vi "simx Set Vision Sensor Image.vi"(5 "operationMode":i32, 6 "options":u8, 7 "bufferSize":i32, 8 "error in (no error)":errorcluster, 9 "image":string, 10 "sensorHandle":i32, 11 "clientID":i32) -> (0 "error out":errorcluster, 1 "image out":string, 3 "function return":i32)   [LabVIEW 2019, in "PXL_V-REP.lvlib"]
doc: "EXTAPI_DLLEXPORT simxInt simxSetVisionSensorImage(simxInt clientID,simxInt sensorHandle,simxUChar* image,simxInt bufferSize,simxUChar options,simxInt operationMode);"
uses:
  PXL_V-REP.lvlib
  <userlib>/V-REP/remoteApi.dll
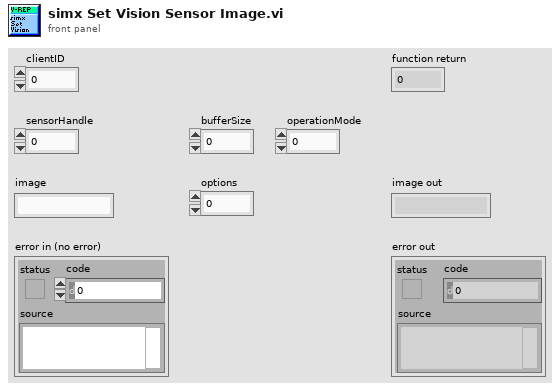
[diagram p1: front panel]
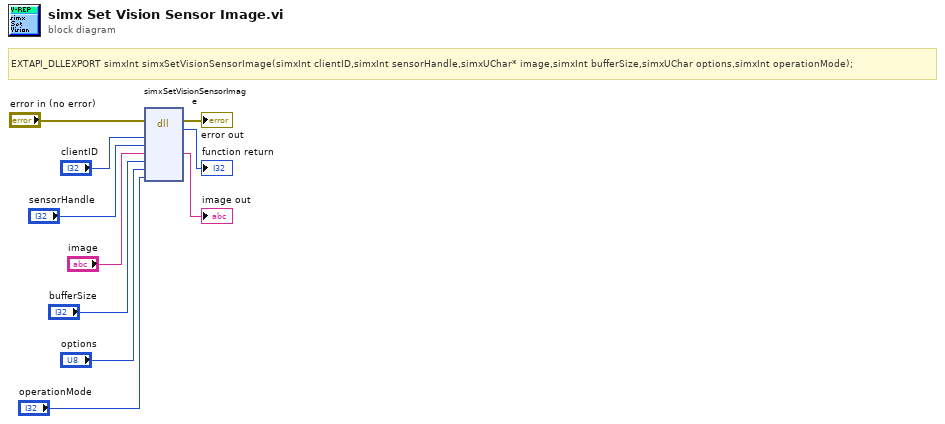
[diagram p0: block diagram]
diagram:
  # "EXTAPI_DLLEXPORT simxInt simxSetVisionSensorImage(simxInt clientID,simxInt sensorHandle,simxUChar* image,simxInt bufferSize,simxUChar options,simxInt operationMode);"
  n1 = dll-call lib="C:/Program Files (x86)/National Instruments/LabVIEW 2019/user.lib/V-REP/remoteApi.*" fn="simxSetVisionSensorImage"(error in="error in (no error)", "clientID"="clientID", "sensorHandle"="sensorHandle", "image"="image", "bufferSize"="bufferSize", "options"="options", "operationMode"="operationMode") -> (error out=→"error out":errorcluster, →"function return":i32, "image"=→"image out":string)  [unwired: 7 in, 1 out]
